vi "Write UI Launched.vi"(10 "Subscriptions.UI Launched":refnum<class "MVC Subscription.lvclass">, 11 "Flex UI (Actor) in":refnum<class "Flex UI (Actor).lvclass">) -> (3 "Flex UI (Actor) out":refnum<class "Flex UI (Actor).lvclass">)   [LabVIEW 2016, in "Flex UI (Parent Actor).lvlib" / "Flex UI (Actor).lvclass"]
uses:
  Flex UI (Actor).lvclass
  <vilib>/East West Architects/MVC Subscription/Subscription/MVC Subscription.lvclass
  Flex UI (Actor).lvclass/Flex UI (Actor).ctl
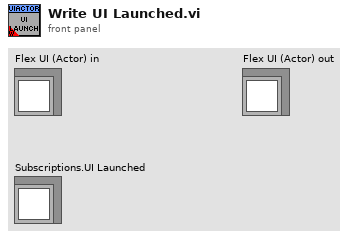
[diagram p1: front panel]
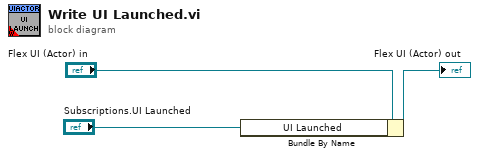
[diagram p0: block diagram]
diagram:
  n1 = Bundle By Name(cluster="Flex UI (Actor) in", "UI Launched"="Subscriptions.UI Launched") -> (→"Flex UI (Actor) out":refnum<class "Flex UI (Actor).lvclass">)
